vi "消息提示.vi"(7 "设置":string[](array[string]), 8 "被测幅值":dbl format="%.2p", 9 "参考幅值":dbl format="%.2p", 10 "参数":string(combo)="参考灵敏度") -> ()   [LabVIEW 2015]
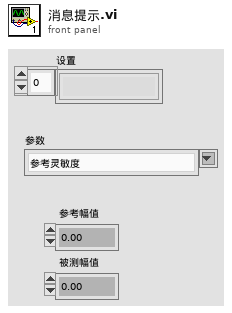
[diagram p1: front panel]
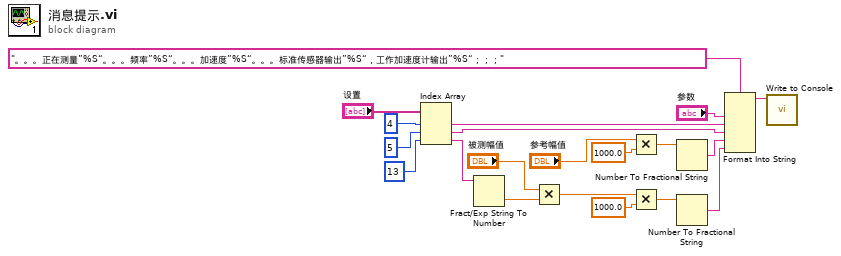
[diagram p0: block diagram]
diagram:
  n1 = Index Array(array="设置", index #1=4 ("索引"), index #2=5 ("索引"), index #3=13 ("索引")) -> (element #1=w16:string, element #2=w6:string, element #3=w7:string)
  n2 = Fract/Exp String To Number(string=w7) -> (number=w13:dbl)  [unwired: 3 in, 1 out]
  n3 = Multiply(x="被测幅值", y=w13) -> (x*y=w12:dbl)
  n4 = Multiply(x="参考幅值", y=1000.0) -> (x*y=w9:dbl)
  n5 = Multiply(x=w12, y=1000.0) -> (x*y=w3:dbl)
  n6 = Number To Fractional String(number=w9) -> (F-format string=w4:string)  [unwired: 3 in]
  n7 = Number To Fractional String(number=w3) -> (F-format string=w2:string)  [unwired: 3 in]
  n8 = Format Into String(format string="。。。正在测量”%S“。。。频率”%S“。。。加速度”%S“。。。标准传感器输出”%S“，工作加速度计输出”%S“；；；" ("分隔符(Tab)"), "参数", w16, w6, w4, w2) -> (resulting string=w1:string)  [unwired: 2 in, 1 out]
  n9 = call "Write to Console.vi"("Input"=w1) -> ()  [unwired: 10 in, 1 out]
